vi "flow_queue_add.vi"(5 "溜まった状態を削除":bool, 7 "前に状態を追加":bool, 8 "error in (no error)":errorcluster caption="エラー入力（エラーなし）", 10 "data":T1, 11 "queue in":refnum<queue>) -> (0 "error out":errorcluster caption="エラー出力", 3 "queue out":refnum<queue>)   [LabVIEW 2017]
uses:
  flow_queue_datatype.ctl
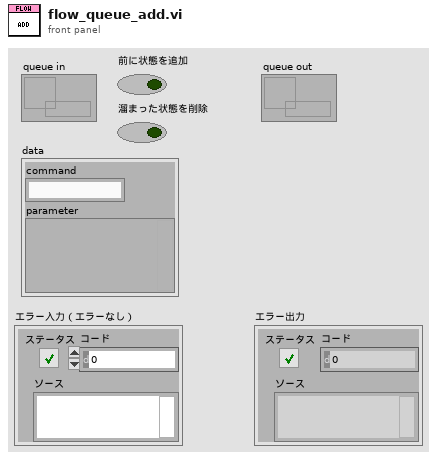
[diagram p1: front panel]
types:
  T1 = typedef "flow_queue_datatype.ctl" = cluster{"command":string, "parameter":variant}
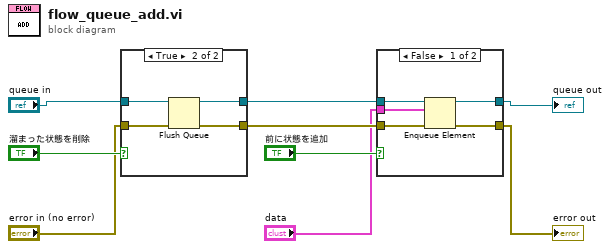
[diagram p0: block diagram]
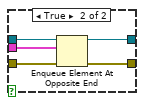
[diagram p2: hidden frame]
diagram:
  n1 = case shown="True" "溜まった状態を削除" {
    tunnel: "queue in" -> [w11 w15]
    tunnel: [w11 w14] -> w7
    tunnel: "error in (no error)" -> [w10 w13]
    tunnel: [w10 w12] -> w4
    frame False {
    }
    frame True {
      n2 = Flush Queue(queue=w15, error in (no error)=w13) -> (queue out=w14:refnum<queue>, error out=w12:errorcluster)  [unwired: 1 out]
    }
  }
  n3 = case shown="False" "前に状態を追加" {
    tunnel: w7 -> [w20 w25]
    tunnel: [w19 w24] -> w5
    tunnel: w4 -> [w17 w23]
    tunnel: [w18 w22] -> w3
    tunnel: "data" -> [w16 w21]
    frame False {
      n4 = Enqueue Element(queue=w20, element=w16, error in (no error)=w17) -> (queue out=w19:refnum<queue>, error out=w18:errorcluster)  [unwired: 1 in, 1 out]
    }
    frame True {
      n5 = Enqueue Element At Opposite End(queue=w25, element=w21, error in (no error)=w23) -> (queue out=w24:refnum<queue>, error out=w22:errorcluster)  [unwired: 1 in, 1 out]
    }
  }
  "error out" <- w3
  "queue out" <- w5
